vi "340 log(SubVI).vi"(11 "Instrument":T2={"325 Resource "="GPIB0::13::INSTR", "Input (0:A) 325"=0, "Heater Output (1:1) 325"=1, "340 Resource"="GPIB0::14::INSTR", "Input (0:A) 340"=0, "Loop (0: 1)"=0, "Input (0:B) 340"=1, "Loop (1: 1)"=2, "340 Status"=refnum, "Instrument Type"=enum."PPMS", "quantum design"=refnum, "semaphore 325"=refnum, "TCP master instance"=refnum, "M24C Resource"="GPIB0::24::INSTR", "4G supply"="GPIB0::24::INSTR", "Temp Status 24C"=refnum, "Temp"=refnum, "9T信号"=refnum, "limit"={"Field limit"=0.0, "Field rate limit"=0.0, "Temp limit"=0.0, "Temp low limit"=0.0, "Temp rate limit "=0.0}, "4g supply status"=refnum, "vi路径"="", "in-plane"="", "out-plane"="", "in-plane signal"=FALSE, "out-plane signal"=FALSE, "in plane 信号"=refnum, "pzt volt"=refnum, "Aborting"=refnum, "数据文件"=refnum, "warning"=refnum, "750 visa"="", "750 rotate"="", "335 Status 2"=refnum, "335 Resource "="GPIB0::24::INSTR", "Input (0:A) 335"=0, "Input (0:B) 335"=1, "Heater Output (1:1) 335"=1, "semaphore 340"=refnum, "semaphore 335"=refnum, "325 Status"=refnum, "semaphore 750"=refnum, "750 field status"=refnum} {"Loop (1: 1)" items=["1"=1, "2"=2]; "Loop (0: 1)" items=["1"=1, "2"=2]; "Input (0:B) 340" items=["A", "B", "C", "D"]; "Heater Output (1:1) 335" items=["1"=1, "2"=2]; "Input (0:B) 335" items=["A", "B"]; "Input (0:A) 335" items=["A", "B"]; "Heater Output (1:1) 325" items=["1"=1, "2"=2]; "Input (0:A) 325" items=["A", "B"]; "Input (0:A) 340" items=["1"=1, "2"=2]}) -> (2 "output cluster":T1)   [LabVIEW 2019, in "Get value.lvlib"]
uses:
  Get value.lvlib
  ctl/Instrument.ctl
  <vilib>/NI/Modbus Library/API/Master/Modbus Master.lvclass
  ctl/335 state.ctl
  ctl/Instrument Type.ctl
  lib/QDInstrument.dll
  ctl/limit.ctl
  ctl/9T mag field stauts.ctl
  ctl/warning.ctl
  lib/Lake Shore 340/Lake Shore Cryotronics 340.lvlib
panel:
  out "error out":errorcluster
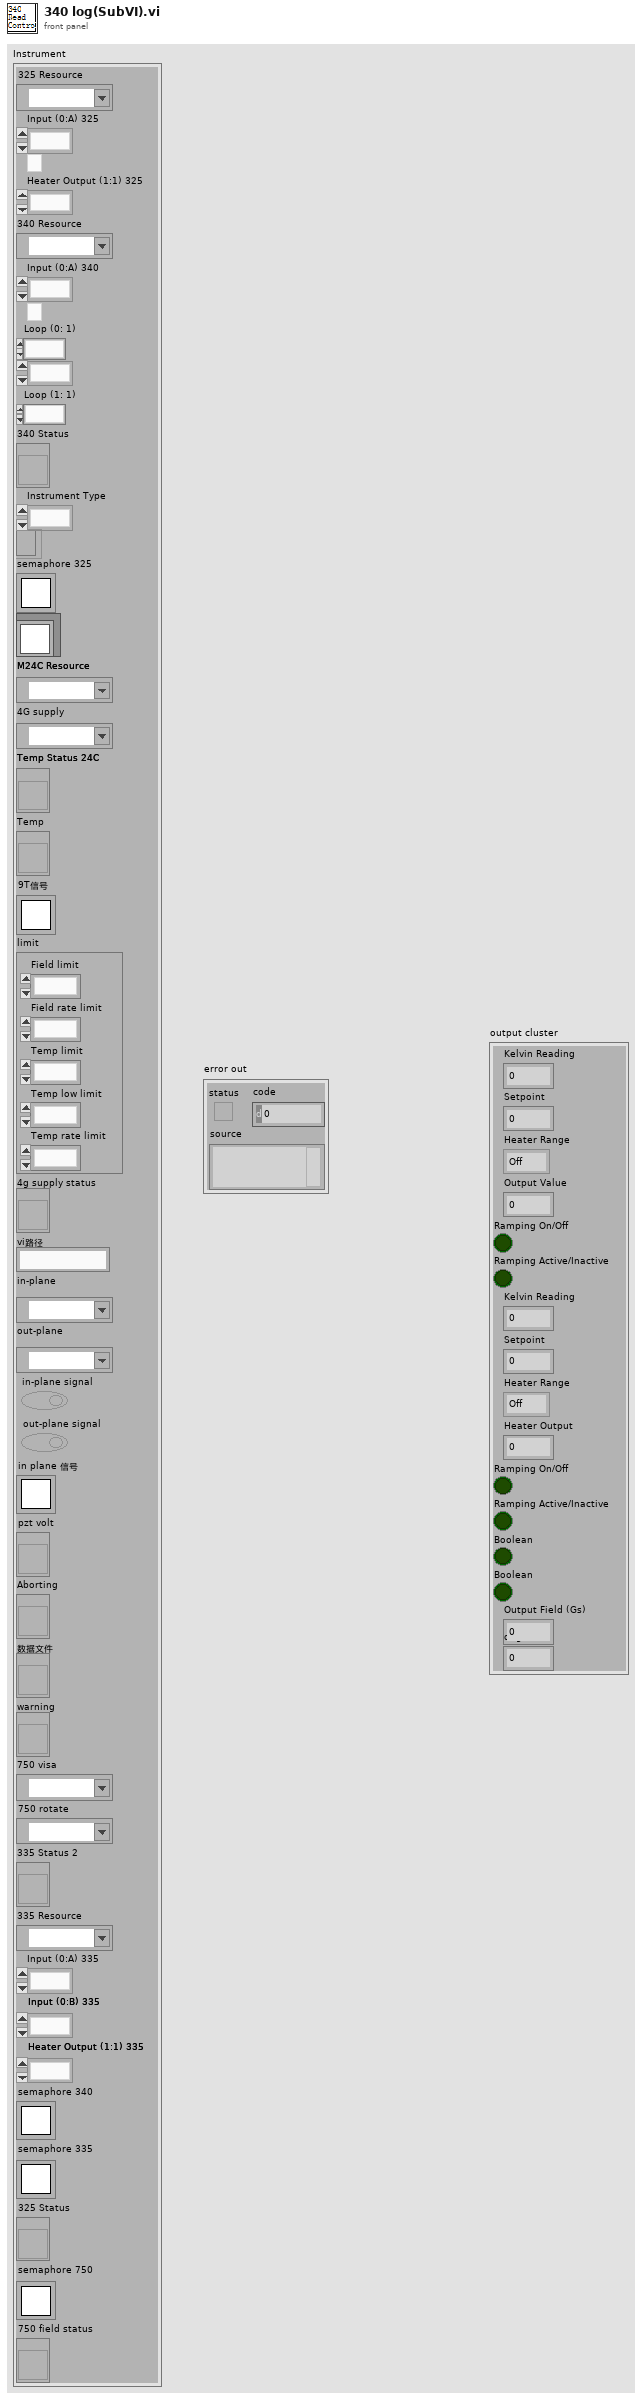
[diagram p1: front panel]
types:
  T1 = cluster{"Kelvin Reading":dbl, "Setpoint":dbl, "Heater Range":enum16{"Off", "On"}, "Output Value":dbl, "Ramping On/Off":bool, "Ramping Active/Inactive":bool, "Kelvin Reading":dbl, "Setpoint":dbl, "Heater Range":enum16{"Off", "1", "2", "3", "4", "5"}, "Heater Output":dbl, "Ramping On/Off":bool, "Ramping Active/Inactive":bool, "Boolean":bool, "Boolean":bool, "Output Field (Gs)":dbl, "degree":dbl}
  T2 = typedef "Instrument.ctl" = cluster{"325 Resource ":refnum<visa-resource-name>, "Input (0:A) 325":u16, "Heater Output (1:1) 325":u16, "340 Resource":refnum<visa-resource-name>, "Input (0:A) 340":u16, "Loop (0: 1)":u16, "Input (0:B) 340":u16, "Loop (1: 1)":u16, "340 Status":refnum<vi>, "Instrument Type":T3, "quantum design":refnum<k24>, "semaphore 325":T4, "TCP master instance":refnum<class "Modbus Master.lvclass">, "M24C Resource":refnum<visa-resource-name>, "4G supply":refnum<visa-resource-name>, "Temp Status 24C":refnum<vi>, "Temp":refnum<vi>, "9T信号":T4, "limit":T5, "4g supply status":refnum<vi>, "vi路径":string, "in-plane":refnum<visa-resource-name>, "out-plane":refnum<visa-resource-name>, "in-plane signal":bool, "out-plane signal":bool, "in plane 信号":T4, "pzt volt":refnum<vi>, "Aborting":refnum<vi>, "数据文件":refnum<vi>, "warning":refnum<vi>, "750 visa":refnum<visa-resource-name>, "750 rotate":refnum<visa-resource-name>, "335 Status 2":refnum<vi>, "335 Resource ":refnum<visa-resource-name>, "Input (0:A) 335":u16, "Input (0:B) 335":u16, "Heater Output (1:1) 335":u16, "semaphore 340":T4, "semaphore 335":T4, "325 Status":refnum<vi>, "semaphore 750":T4, "750 field status":refnum<vi>}
  T3 = typedef "Instrument Type.ctl" = enum16{"PPMS", "VersaLab", "DynaCool", "SVSM", "PPMS-Rotate", "Lakeshore335", "lengtou2", "9T mag", "9T cmag rotate", "test"}
  T4 = typedef "Semaphore RefNum" = refnum<k1>
  T5 = typedef "limit.ctl" = cluster{"Field limit":dbl, "Field rate limit":dbl, "Temp limit":dbl, "Temp low limit":dbl, "Temp rate limit ":dbl}
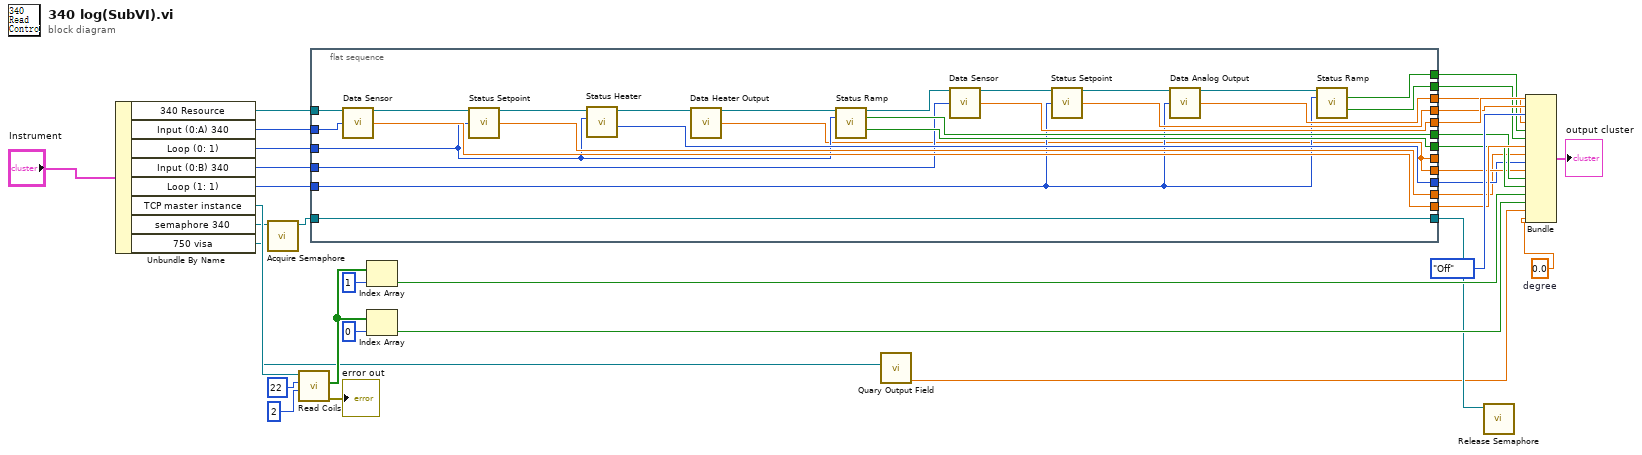
[diagram p0: block diagram]
diagram:
  w3 = 0.0  # degree
  n1 = Unbundle By Name("Instrument") -> ("340 Resource"=w23:refnum<visa-resource-name>, "Input (0:A) 340"=w22:u16, "Loop (0: 1)"=w21:u16, "Input (0:B) 340"=w20:u16, "Loop (1: 1)"=w19:u16, "TCP master instance"=w27:refnum<class "Modbus Master.lvclass">, "semaphore 340"=w26:T4, "750 visa"=w2:refnum<visa-resource-name>)
  n2 = call <vilib>:"Acquire Semaphore.vi"("semaphore"=w26) -> ("semaphore out"=w12:T4)  [unwired: 4 in, 2 out]
  n3 = call-dynamic "Read Coils.vi"("number of inputs"=u16 2, "starting address"=u16 22, "Modbus master in"=w27) -> ("error out"=→"error out":errorcluster, "coils"=w34:bool[])  [unwired: 6 in, 1 out]
  n4 = flat-sequence {
    tunnel: [w56] -> w5
    tunnel: w23 -> [w58]
    tunnel: w12 -> [w59]
    tunnel: [w59] -> w11
    tunnel: w22 -> [w48]
    tunnel: [w57] -> w8
    tunnel: [w55] -> w10
    tunnel: [w53] -> w9
    tunnel: [w35] -> _
    tunnel: w21 -> [w38]
    tunnel: [w49] -> w6
    tunnel: [w47] -> w18
    tunnel: w20 -> [w45]
    tunnel: [w42] -> w17
    tunnel: [w41] -> w13
    tunnel: [w40] -> w15
    tunnel: [w39] -> w14
    tunnel: w19 -> [w37]
    tunnel: [w35] -> w7
    frame #0 {
      n5 = call "Data Sensor.vi"("VISA resource name"=w58, "Input (0: A)"=w48) -> ("VISA resource name out"=w54:refnum<visa-resource-name>, "Kelvin Reading"=w55:dbl)  [unwired: 9 in, 3 out]
      n6 = call "Status Setpoint.vi"("VISA resource name"=w54, "Loop (0: 1)"=w38) -> ("VISA resource name out"=w51:refnum<visa-resource-name>, "Setpoint"=w56:dbl)  [unwired: 11 in, 1 out]
      n7 = call "Status Heater.vi"("Loop"=w38, "VISA resource name"=w51) -> ("Heater Range"=w49:enum16{"Off", "1", "2", "3", "4", "5"}, "VISA resource name out"=w50:refnum<visa-resource-name>)  [unwired: 7 in, 1 out]
      n8 = call "Data Heater Output.vi"("VISA resource name"=w50) -> ("VISA resource name out"=w52:refnum<visa-resource-name>, "Heater Output"=w35:dbl)  [unwired: 12 in, 1 out]
      n9 = call "Status Ramp.vi"("VISA resource name"=w52, "Loop (0: 1)"=w38) -> ("VISA resource name out"=w46:refnum<visa-resource-name>, "Ramping On/Off"=w53:bool, "Ramping Active/Inactive"=w57:bool)  [unwired: 9 in, 2 out]
      n10 = call "Data Sensor.vi"("VISA resource name"=w46, "Input (0: A)"=w45) -> ("VISA resource name out"=w44:refnum<visa-resource-name>, "Kelvin Reading"=w47:dbl)  [unwired: 9 in, 3 out]
      n11 = call "Status Setpoint.vi"("VISA resource name"=w44, "Loop (0: 1)"=w37) -> ("VISA resource name out"=w36:refnum<visa-resource-name>, "Setpoint"=w42:dbl)  [unwired: 11 in, 1 out]
      n12 = call "Data Analog Output.vi"("VISA resource name"=w36, "Analog Output (0: 1)"=w37) -> ("VISA resource name out"=w43:refnum<visa-resource-name>, "Output Value"=w41:dbl)  [unwired: 11 in, 1 out]
      n13 = call "Status Ramp.vi"("VISA resource name"=w43, "Loop (0: 1)"=w37) -> ("Ramping On/Off"=w40:bool, "Ramping Active/Inactive"=w39:bool)  [unwired: 9 in, 3 out]
    }
  }
  n14 = Index Array(array=w34, index=1) -> (element=w24:bool)
  n15 = Index Array(array=w34, index=0) -> (element=w25:bool)
  n16 = call "Quary Output Field.vi"("VISA resource name"=w2) -> ("Output Field (Gs)"=w4:dbl)  [unwired: 8 in, 2 out]
  n17 = call <vilib>:"Release Semaphore.vi"("semaphore"=w11) -> ()  [unwired: 5 in, 2 out]
  n18 = Bundle("Kelvin Reading"=w18, "Setpoint"=w17, "Heater Range"=enum16{"Off", "On"}."Off", "Output Value"=w13, "Ramping On/Off"=w15, "Ramping Active/Inactive"=w14, "Kelvin Reading"=w10, "Setpoint"=w5, "Heater Range"=w6, "Heater Output"=w7, "Ramping On/Off"=w9, "Ramping Active/Inactive"=w8, "Boolean"=w24, "Boolean"=w25, "Output Field (Gs)"=w4, "degree"=w3) -> (→"output cluster":T1)  [unwired: 1 in]
